vi "DriveSliceThreshold(SubVI).vi"(9 "RampValue":dbl, 10 "Motor Power":dbl, 11 "Joystick":dbl) -> (3 "Boolean":bool)   [LabVIEW 2014]
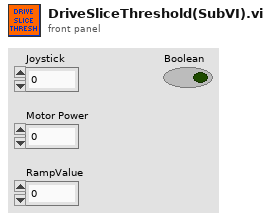
[diagram p1: front panel]
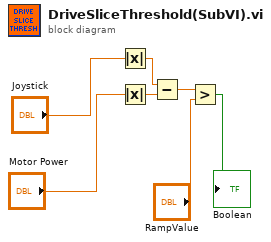
[diagram p0: block diagram]
diagram:
  n1 = Absolute Value(x="Joystick") -> (abs(x)=w2:dbl)
  n2 = Absolute Value(x="Motor Power") -> (abs(x)=w4:dbl)
  n3 = Subtract(x=w2, y=w4) -> (x-y=w1:dbl)
  n4 = Greater?(x=w1, y="RampValue") -> (0:→"Boolean":bool)
